vi "TestPanel.vi"() -> ()   [LabVIEW 2014]
panel:
  in  "Reset":bool
  in  "Levitation":bool
  in  "SensePwr":bool
  in  "ToF 8":bool
  in  "ToF 7":bool
  in  "ToF 6":bool
  in  "ToF 5":bool
  in  "ToF 4":bool
  in  "ToF 3":bool
  in  "ToF 2":bool
  in  "ToF 1":bool
  in  "stop":bool
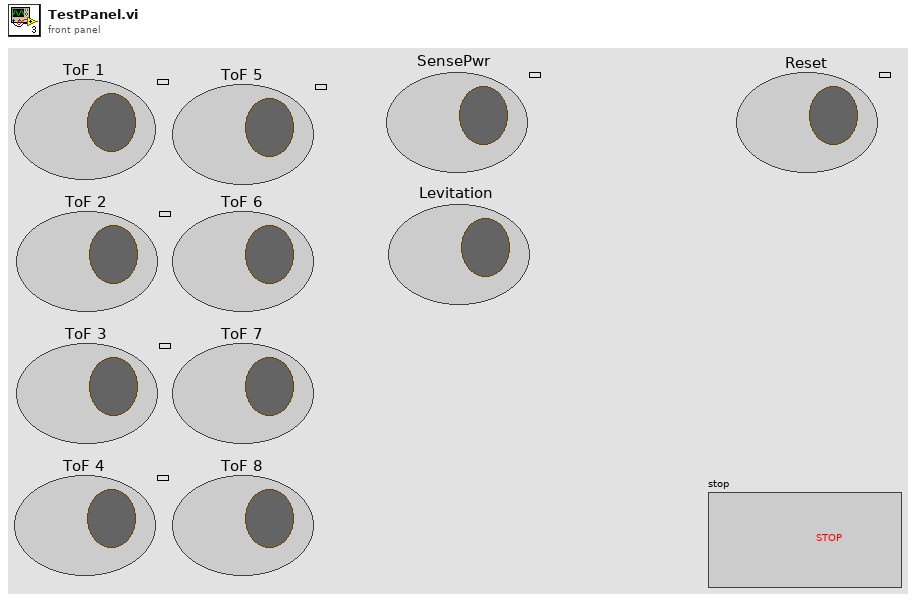
[diagram p1: front panel]
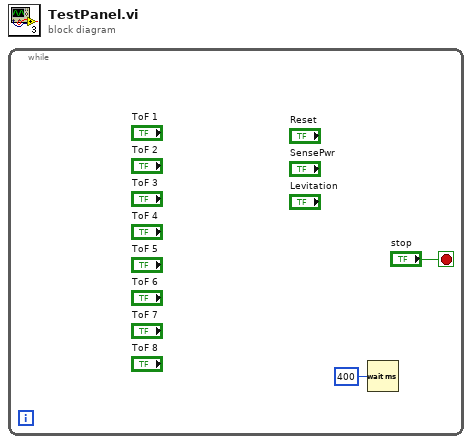
[diagram p0: block diagram]
diagram:
  n1 = while {
    stop <- "stop" stop-if-true
    n2 = Wait (ms)(milliseconds to wait=u32 400) -> ()  [unwired: 1 out]
  }
